vi "Conv_Deg_Rotations.vi"(10 "Degrees":dbl) -> (2 "Rotations":dbl)   [LabVIEW 2019, in "Trajectory_Library.lvlib"]
doc: "Convert Degrees to Rotations"
uses:
  Trajectory_Library.lvlib
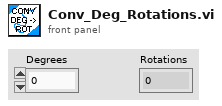
[diagram p1: front panel]
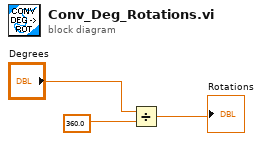
[diagram p0: block diagram]
diagram:
  n1 = Divide(x="Degrees", y=360.0) -> (x/y=→"Rotations":dbl)
